vi "WeatherMapAPI_CurrentWeather-ConvertUtcTimeToStrings.vi"(7 "1Hr Adjust - Subtract":bool, 9 "Offset from UTC":string, 11 "Sunrise/Sunset time, unix, UTC":string) -> (1 "Date":string, 3 "Time":string)   [LabVIEW 2021]
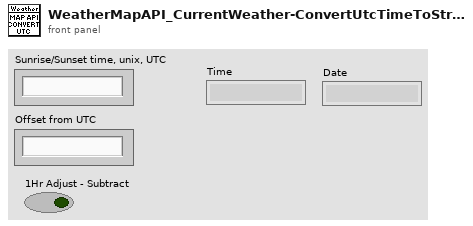
[diagram p1: front panel]
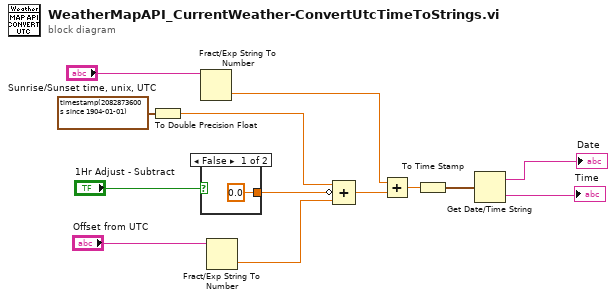
[diagram p0: block diagram]
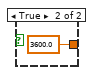
[diagram p2: hidden frame]
diagram:
  n1 = To Double Precision Float(number=timestamp(2082873600 s since 1904-01-01) ("time stamp")) -> (double precision float=w8:dbl)
  n2 = Fract/Exp String To Number(string="Sunrise/Sunset time, unix, UTC") -> (number=w3:dbl)  [unwired: 3 in, 1 out]
  n3 = case shown="False" "1Hr Adjust - Subtract" {
    tunnel: [0.0 ("number") 3600.0 ("number")] -> w7
    frame False {
    }
    frame True {
    }
  }
  n4 = Fract/Exp String To Number(string="Offset from UTC") -> (number=w1:dbl)  [unwired: 3 in, 1 out]
  n5 = Compound Arithmetic op=ADD(w8, invert w7, w1) -> (w5:dbl)
  n6 = Add(x=w3, y=w5) -> (x+y=w9:dbl)
  n7 = To Time Stamp(1:w9) -> (0:w10:timestamp)
  n8 = Get Date/Time String(seconds (now)=w10) -> (date string=→"Date":string, time string=→"Time":string)  [unwired: 2 in]
